vi "test_easy_linear_vs_spline_interpl.vi"() -> ()   [LabVIEW 2009]
doc: "Copyright (C) 2009, Stepan A. Baranov\nweb: http://www.OCTLab.org/\nemail: stepan@baranov.su"
uses:
  <vilib>/Analysis/NI_AALPro.lvlib
  OCTLib.dll
panel:
  out "error out":errorcluster
  in  "Small/Big":bool
  out "XY Graph":cluster{"Y":dbl[], "Y":dbl[]}[](graph)
  out "Waveform Graph":dbl[][](graph)
  out "width":i32
  out "height":i32
  out "loop #":i32
  out "RSM_STAT time":u32
  out "LabView time":u32
  out "RSM_STAT Array":dbl[][](array[numeric])
  out "LabView Array":dbl[][](array[numeric])
  in  "stop":bool
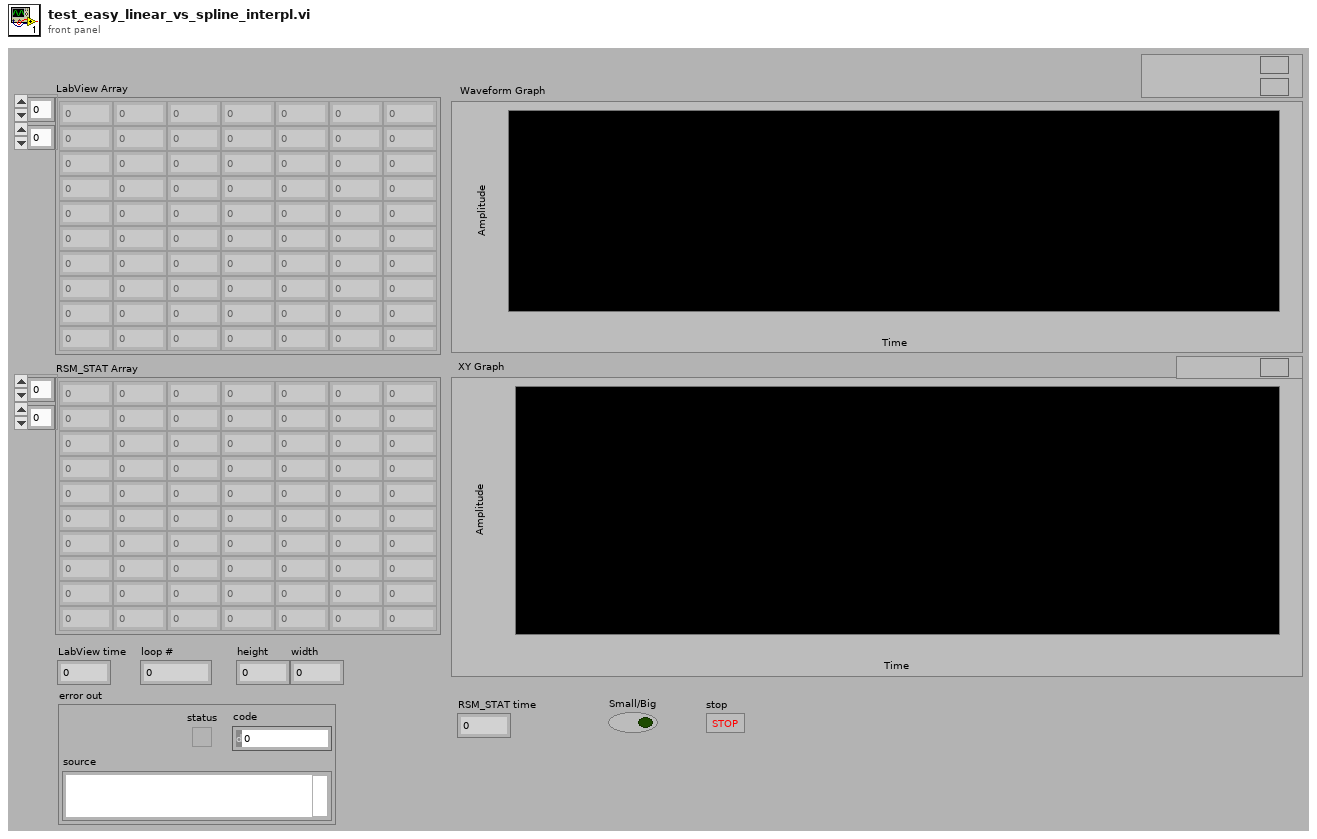
[diagram p1: front panel]
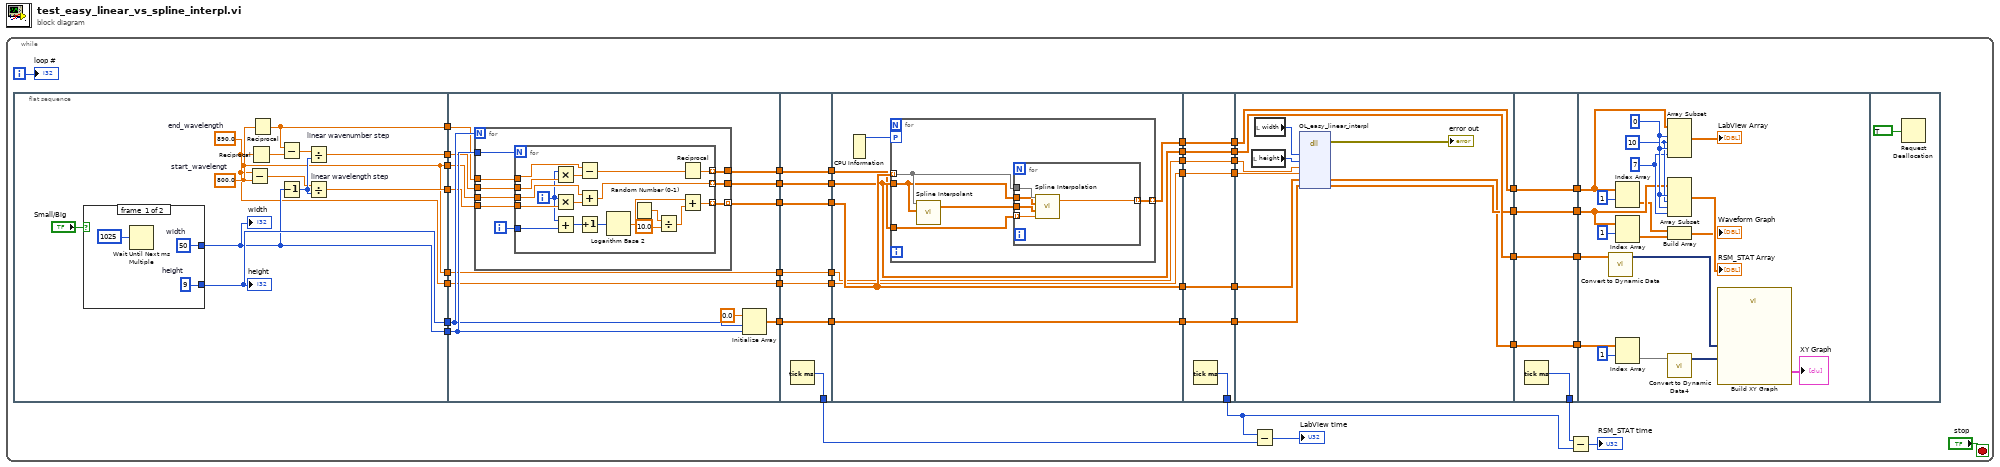
[diagram p0: block diagram]
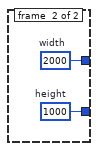
[diagram p2: hidden frame]
diagram:
  n1 = while {
    i -> [w41]
    stop <- "stop" stop-if-true
    n2 = flat-sequence {
      tunnel: [w54] -> w38
      tunnel: [w59] -> w37
      tunnel: [w53] -> w14
      tunnel: [w49] -> w13
      tunnel: [w52] -> w12
      tunnel: [w51] -> w11
      tunnel: [w49] -> w6
      tunnel: [w48] -> w1
      tunnel: [w73] -> w39
      tunnel: w38 -> [w72]
      tunnel: w37 -> [w71]
      tunnel: [w74] -> w36
      tunnel: [w76] -> w33
      tunnel: [w75] -> w28
      tunnel: w14 -> [w70]
      tunnel: w13 -> [w69]
      tunnel: w12 -> [w68]
      tunnel: w11 -> [w67]
      tunnel: [w66] -> w7
      tunnel: w6 -> [w66]
      tunnel: [w65] -> w2
      tunnel: w1 -> [w65]
      tunnel: [w111] -> w46
      tunnel: [w110] -> w40
      tunnel: w39 -> [w110]
      tunnel: w36 -> [w109]
      tunnel: [w109] -> w35
      tunnel: [w108] -> w34
      tunnel: w33 -> [w108]
      tunnel: w28 -> [w107]
      tunnel: [w107] -> w27
      tunnel: [w106] -> w8
      tunnel: w7 -> [w106]
      tunnel: [w105] -> w3
      tunnel: w2 -> [w105]
      tunnel: w40 -> [w117]
      tunnel: w35 -> [w118]
      tunnel: w34 -> [w116]
      tunnel: [w118] -> w31
      tunnel: [w117] -> w29
      tunnel: w27 -> [w115]
      tunnel: [w115] -> w26
      tunnel: [w114] -> w15
      tunnel: [w113] -> w9
      tunnel: w8 -> [w113]
      tunnel: [w112] -> w4
      tunnel: w3 -> [w112]
      tunnel: [w136] -> w43
      tunnel: [w135] -> w32
      tunnel: w31 -> [w135]
      tunnel: [w134] -> w30
      tunnel: w29 -> [w134]
      tunnel: w26 -> [w133]
      tunnel: [w133] -> w25
      tunnel: [w132] -> w16
      tunnel: w15 -> [w132]
      tunnel: [w131] -> w10
      tunnel: w9 -> [w131]
      tunnel: [w130] -> w5
      tunnel: w4 -> [w130]
      tunnel: w32 -> [w143]
      tunnel: w30 -> [w142]
      tunnel: w25 -> [w145]
      tunnel: [w137] -> w23
      tunnel: [w142] -> w21
      tunnel: [w141] -> w19
      tunnel: [w140] -> w17
      tunnel: w16 -> [w140]
      tunnel: w10 -> [w139]
      tunnel: w5 -> [w138]
      tunnel: [w152] -> w44
      tunnel: [w151] -> w24
      tunnel: w23 -> [w151]
      tunnel: [w150] -> w22
      tunnel: w21 -> [w150]
      tunnel: [w149] -> w20
      tunnel: w19 -> [w149]
      tunnel: [w148] -> w18
      tunnel: w17 -> [w148]
      tunnel: w24 -> [w159]
      tunnel: w22 -> [w158]
      tunnel: w20 -> [w157]
      tunnel: w18 -> [w156]
      frame #0 {
        w49 = 800.0  # start_wavelengt
        w48 = 890.0  # end_wavelength
        n3 = case shown="False" "Small/Big" {
          tunnel: [w62 w63] -> w59
          tunnel: [w61 w64] -> w54
          frame #0 {
            w61 = 50  # width
            w62 = 9  # height
            n4 = Wait Until Next ms Multiple(millisecond multiple=u32 1025) -> ()  [unwired: 1 out]
          }
          frame #1 {
            w64 = 2000  # width
            w63 = 1000  # height
          }
        }
        "height" <- w59
        "width" <- w54
        n5 = Subtract(x=w48, y=w49) -> (x-y=w50:dbl)
        n6 = Reciprocal(x=w48) -> (1/x=w55:dbl)
        n7 = Reciprocal(x=w49) -> (1/x=w51:dbl)
        n8 = Subtract(x=w51, y=w55) -> (x-y=w57:dbl)
        n9 = Decrement(x=w54) -> (x-1=w56:i32)
        n10 = Divide "linear wavenumber step"(x=w57, y=w56) -> (x/y=w52:dbl)
        n11 = Divide "linear wavelength step"(x=w50, y=w56) -> (x/y=w53:dbl)
      }
      frame #1 {
        n12 = for {
          N: w71 -> [_]
          tunnel: w72 -> [w86]
          tunnel: [w85] -> w73
          tunnel: [w84] -> w74 mode=indexing
          tunnel: [w83] -> w76
          tunnel: w70 -> [w82]
          tunnel: w69 -> [w81]
          tunnel: w68 -> [w80]
          tunnel: w67 -> [w79]
          i -> [w78]
          n13 = for {
            N: w86 -> [_]
            tunnel: [w99] -> w85 mode=indexing
            tunnel: [w87] -> w84 mode=indexing
            tunnel: [w96] -> w83 mode=indexing
            tunnel: w82 -> [w101]
            tunnel: w81 -> [w100]
            tunnel: w80 -> [w98]
            tunnel: w79 -> [w97]
            tunnel: w78 -> [w88]
            i -> [w89]
            n14 = Multiply(x=w89, y=w98) -> (x*y=w104:dbl)
            n15 = Multiply(x=w89, y=w101) -> (x*y=w103:dbl)
            n16 = Add(x=w89, y=w88) -> (x+y=w95:i32)
            n17 = Subtract(x=w97, y=w104) -> (x-y=w102:dbl)
            n18 = Add(x=w100, y=w103) -> (x+y=w99:dbl)
            n19 = Increment(x=w95) -> (x+1=w94:i32)
            n20 = Logarithm Base 2(1:w94) -> (0:w93:dbl)
            n21 = Random Number (0-1)() -> (number: 0 to 1=w92:dbl)
            n22 = Divide(x=w92, y=10.0) -> (x/y=w90:dbl)
            n23 = Reciprocal(x=w102) -> (1/x=w96:dbl)
            n24 = Add(x=w93, y=w90) -> (x+y=w87:dbl)
          }
        }
        n25 = Initialize Array(0.0 ("element"), w71, w72) -> (w75:dbl[][])
      }
      frame #2 {
        n26 = Tick Count (ms)() -> (millisecond timer value=w111:u32)
      }
      frame #3 {
        n27 = CPU Information() -> (4:w119:i32)  [unwired: 3 out]
        n28 = for {
          tunnel: w117 -> [w122]
          workers-P: w119 -> [_]
          tunnel: w118 -> [w123] mode=indexing
          tunnel: w116 -> [w121]
          tunnel: [w120] -> w114 mode=indexing
          n29 = call <vilib>:"Spline Interpolant.vi"("X"=w122, "Y"=w123) -> ("Interpolant"=w124:dbl[])  [unwired: 2 in, 1 out]
          n30 = for {
            tunnel: w124 -> [w129]
            tunnel: w123 -> [w128]
            tunnel: w122 -> [w127]
            tunnel: w121 -> [w126] mode=indexing
            tunnel: [w125] -> w120 mode=indexing
            n31 = call <vilib>:"Spline Interpolation.vi"("x value"=w126, "Interpolant"=w129, "X"=w127, "Y"=w128) -> ("interpolation value"=w125:dbl)  [unwired: 1 out]
          }
        }
      }
      frame #4 {
        n32 = Tick Count (ms)() -> (millisecond timer value=w136:u32)
      }
      frame #5 {
        n33 = local read "height"() -> (w146:i32)
        n34 = local read "width"() -> (w147:i32)
        n35 = dll-call lib="OCTLib.dll" fn="OL_easy_linear_interpl"("width"=w147, "height"=w146, "start_wavelength"=w139, "end_wavelength"=w138, "in"=w143, "out"=w145) -> (error out=→"error out":errorcluster, "in"=w137:dbl[][], "out"=w141:dbl[][])  [unwired: 8 in, 1 out]
      }
      frame #6 {
        n36 = Tick Count (ms)() -> (millisecond timer value=w152:u32)
      }
      frame #7 {
        w170 = 10 ("length")
        w169 = 7 ("length")
        w171 = 0 ("index")
        n37 = call "Convert to Dynamic Data"("Array"=w158) -> ("Dynamic Data Type"=w161:dynamicdata)  [unwired: 3 in]
        n38 = Index Array(array=w156, index (row)=1) -> (element=w155:dbl[])  [unwired: 1 in]
        n39 = Index Array(array=w157, index (row)=1) -> (element=w154:dbl[])  [unwired: 1 in]
        n40 = Index Array(array=w159, index (row)=1) -> (element=w163:dbl[])  [unwired: 1 in]
        n41 = Array Subset(array=w156, index (row)=w171, length (row)=w170, index (col)=w171, length (col)=w169) -> (→"LabView Array":dbl[][])
        n42 = Array Subset(array=w157, index (row)=w171, length (row)=w170, index (col)=w171, length (col)=w169) -> (→"RSM_STAT Array":dbl[][])
        n43 = Build Array(w155, w154) -> (→"Waveform Graph":dbl[][])
        n44 = call "Convert to Dynamic Data4"("Array"=w163) -> ("Dynamic Data Type"=w162:dynamicdata)  [unwired: 3 in]
        n45 = call "Build XY Graph"("Y Input"=w162, "X Input"=w161) -> ("XY Graph"=→"XY Graph":cluster{"Y":dbl[], "Y":dbl[]}[])  [unwired: 8 in, 1 out]
      }
      frame #8 {
        n46 = Request Deallocation(TRUE ("flag")) -> ()
      }
    }
    n47 = Subtract(x=w43, y=w46) -> (x-y=→"LabView time":u32)
    n48 = Subtract(x=w44, y=w43) -> (x-y=→"RSM_STAT time":u32)
    "loop #" <- w41
  }
